vi "If IfElse and Switch Statements.vi"() -> ()   [LabVIEW 2015]
panel:
  out "User Output Multiplied":i8
  out "If-Else Numeric Output":i8
  out "\"If-Else\" String Indicator":string
  out "Random Number":i8
  out "\"If\" String Indicator":string
  out "String Output":string
  in  "User Input":i8
  # "If with Select Function"
  # "If with Case Structure"
  # "If Else / Switch with Case Structure"
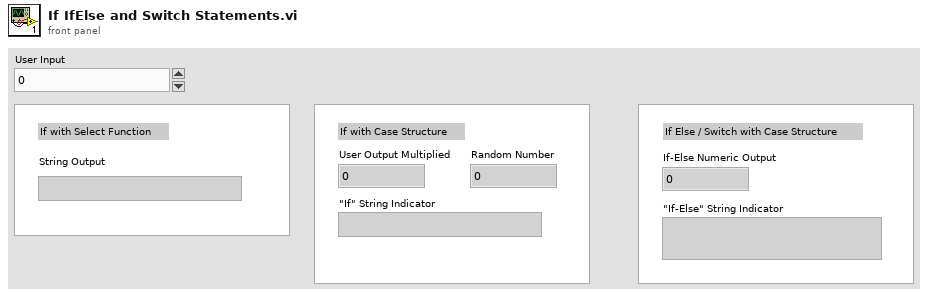
[diagram p1: front panel]
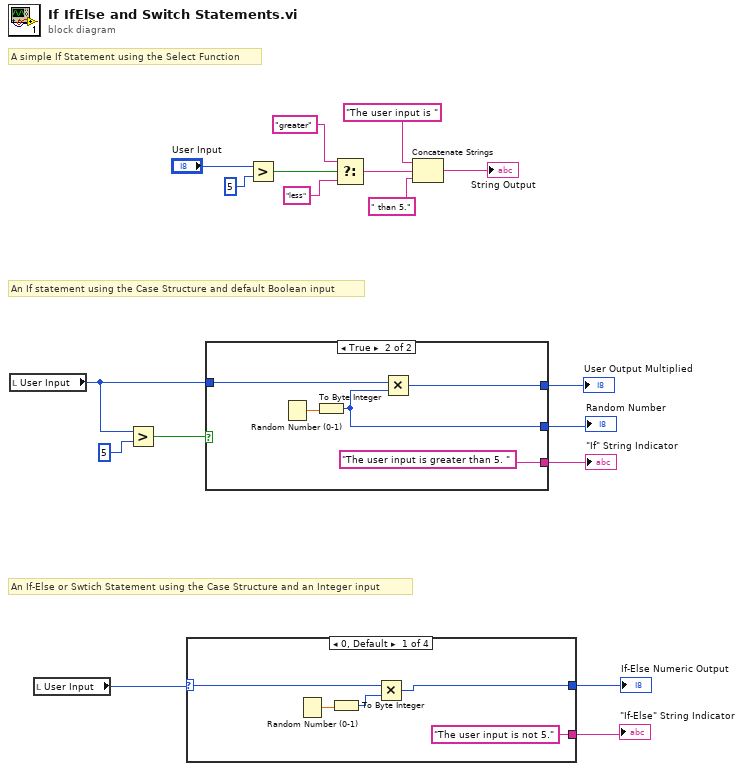
[diagram p0: block diagram]
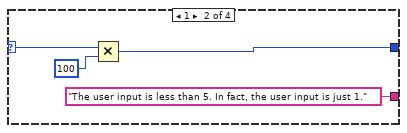
[diagram p2: hidden frame]
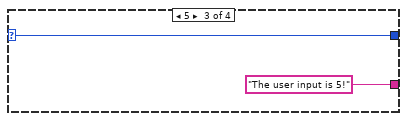
[diagram p3: hidden frame]
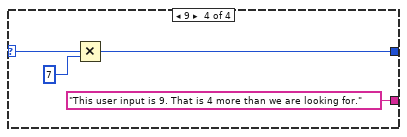
[diagram p4: hidden frame]
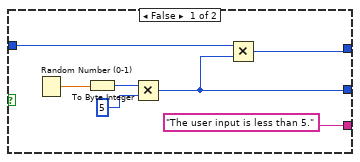
[diagram p5: hidden frame]
diagram:
  # "An If-Else or Swtich Statement using the Case Structure and an Integer input"
  # "An If statement using the Case Structure and default Boolean input"
  # "A simple If Statement using the Select Function"
  n1 = local read "User Input"() -> (w8:i8)
  n2 = local read "User Input"() -> (w7:i8)
  n3 = Greater?(x=w8, y=i8 5) -> (0:w10:bool)
  n4 = case shown="0, Default" w7 {
    selector: w7 -> [w20 w26 w28 w32]
    tunnel: ["The user input is not 5." ("string") "The user input is less than 5. In fact, the user input is just 1." ("string") "The user input is 5!" ("string") "This user input is 9. That is 4 more than we are looking for." ("string")] -> w3
    tunnel: [w19 w24 w28 w30] -> w2
    frame 0, Default {
      n5 = Random Number (0-1)() -> (number: 0 to 1=w21:dbl)
      n6 = To Byte Integer(number=w21) -> (8bit integer=w22:i8)
      n7 = Multiply(x=w20, y=w22) -> (x*y=w19:i8)
    }
    frame 1 {
      n8 = Multiply(x=w26, y=i8 100) -> (x*y=w24:i8)
    }
    frame 5 {
    }
    frame 9 {
      n9 = Multiply(x=w32, y=i8 7) -> (x*y=w30:i8)
    }
  }
  "\"If-Else\" String Indicator" <- w3
  "If-Else Numeric Output" <- w2
  n10 = case shown="True" w10 {
    tunnel: ["The user input is less than 5." ("string") "The user input is greater than 5. " ("string")] -> w9
    tunnel: w8 -> [w40 w44]
    tunnel: [w34 w41] -> w4
    tunnel: [w35 w43] -> w1
    frame False {
      n11 = Random Number (0-1)() -> (number: 0 to 1=w38:dbl)
      n12 = To Byte Integer(number=w38) -> (8bit integer=w37:i8)
      n13 = Multiply(x=w37, y=i8 5) -> (x*y=w34:i8)
      n14 = Multiply(x=w40, y=w34) -> (x*y=w35:i8)
    }
    frame True {
      n15 = Random Number (0-1)() -> (number: 0 to 1=w42:dbl)
      n16 = To Byte Integer(number=w42) -> (8bit integer=w41:i8)
      n17 = Multiply(x=w44, y=w41) -> (x*y=w43:i8)
    }
  }
  "\"If\" String Indicator" <- w9
  "Random Number" <- w4
  "User Output Multiplied" <- w1
  n18 = Greater?(x="User Input", y=i8 5) -> (0:w16:bool)
  n19 = Select(t="greater", s=w16, f="less") -> (s? t:f=w14:string)
  n20 = Concatenate Strings "Concatenate Strings"("The user input is " ("string"), w14, " than 5." ("string")) -> (→"String Output":string)
